vi "start.vi"(8 "error in (no error)":errorcluster, 10 "Model in":refnum<class "Model.lvclass">, 11 "StandbyState in":refnum<class "StandbyState.lvclass">) -> (0 "error out":errorcluster, 2 "Model out":refnum<class "Model.lvclass">, 3 "StandbyState out":refnum<class "StandbyState.lvclass">)   [LabVIEW 2015, in "StandbyState.lvclass"]
uses:
  StandbyState.lvclass
  Typedefs/StateSelector.ctl
  Typedefs/FAMTTypedefs.lvlib
  Model/Model/Model.lvclass
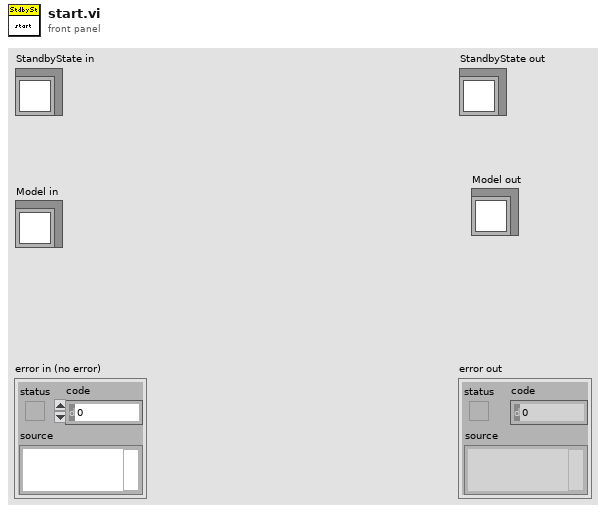
[diagram p1: front panel]
types:
  T1 = typedef "FAMTTypedefs.lvlib/StateSelector.ctl" = enum16{"OfflineState", "FaultState", "StandbyState", "DisabledState", "EnabledState", "WaitForUserInputState", "PerformOpenLoopScanState", "PerformPreScanHoldState", "PerformPostScanHoldState", "PerformScanState"}
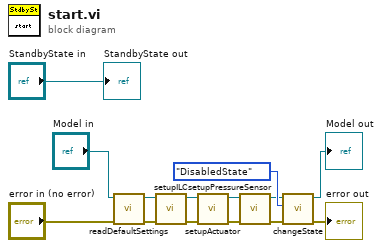
[diagram p0: block diagram]
diagram:
  n1 = call "readDefaultSettings.vi"("error in (no error)"="error in (no error)", "Model in"="Model in") -> ("error out"=w3:errorcluster, "Model out"=w2:refnum<class "Model.lvclass">)  [unwired: 8 in]
  n2 = call "setupILC.vi"("error in (no error)"=w3, "Model in"=w2) -> ("error out"=w8:errorcluster, "Model out"=w11:refnum<class "Model.lvclass">)  [unwired: 8 in]
  n3 = call "setupActuator.vi"("error in (no error)"=w8, "Model in"=w11) -> ("error out"=w7:errorcluster, "Model out"=w10:refnum<class "Model.lvclass">)  [unwired: 8 in]
  n4 = call "setupPressureSensor.vi"("error in (no error)"=w7, "Model in"=w10) -> ("error out"=w6:errorcluster, "Model out"=w9:refnum<class "Model.lvclass">)  [unwired: 8 in]
  n5 = call "changeState.vi"("error in (no error)"=w6, "State:"=StateSelector."DisabledState", "Model in"=w9) -> ("error out"=→"error out":errorcluster, "Model out"=→"Model out":refnum<class "Model.lvclass">)  [unwired: 7 in]
  "StandbyState out" <- "StandbyState in"
